vi "Set Description.vi"(8 "error in":errorcluster, 10 "Description":string, 11 "Sub Object in":refnum<class "Sub Object.lvclass">) -> (0 "error out":errorcluster, 3 "Sub Object out":refnum<class "Sub Object.lvclass">)   [LabVIEW 2020, in "CANopen.lvlib" / "Sub Object.lvclass"]
uses:
  Sub Object.lvclass
  Sub Object.lvclass/Sub Object.ctl
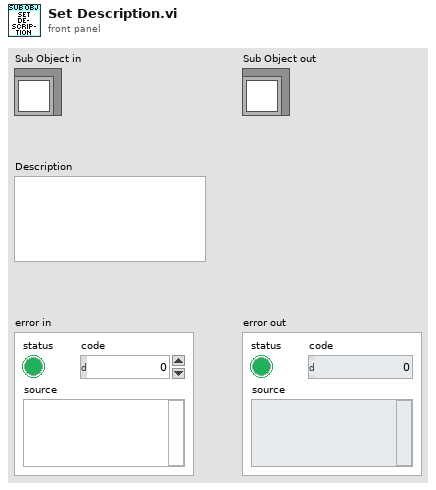
[diagram p1: front panel]
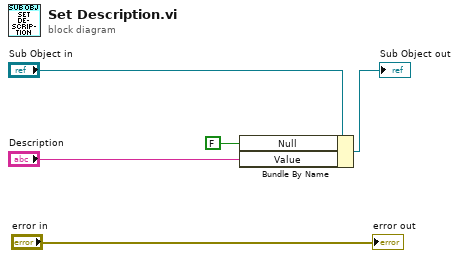
[diagram p0: block diagram]
diagram:
  n1 = Bundle By Name(cluster="Sub Object in", "Null"=FALSE ("Description.Null"), "Value"="Description") -> (→"Sub Object out":refnum<class "Sub Object.lvclass">)
  "error out" <- "error in"
